vi "mobileye_disp.vi"(11 "x_view":dbl[](array[numeric])=[0.0, 0.5, 1.0, 1.5, 2.0, 2.5, 3.0, 3.5, 4.0, 4.5, 5.0, 5.5, 6.0, 6.5, 7.0, 7.5, 8.0, 8.5, 9.0, 9.5, 10.0, 10.5, 11.0, 11.5, 12.0, 12.5, 13.0, 13.5, 14.0, 14.5, 15.0, 15.5, 16.0, 16.5, 17.0, 17.5, 18.0, 18.5, 19.0, 19.5, 20.0, 20.5, 21.0, 21.5, 22.0, 22.5, 23.0, 23.5, 24.0, 24.5, 25.0, 25.5, 26.0, 26.5, 27.0, 27.5, 28.0, 28.5, 29.0, 29.5, 30.0, 30.5, 31.0, 31.5, 32.0, 32.5, 33.0, 33.5, 34.0, 34.5, 35.0, 35.5, 36.0, 36.5, 37.0, 37.5, 38.0, 38.5, 39.0, 39.5, 40.0, 40.5, 41.0, 41.5, 42.0, 42.5, 43.0, 43.5, 44.0, 44.5, 45.0, 45.5, 46.0, 46.5, 47.0, 47.5, 48.0, 48.5, 49.0, 49.5, 50.0, 50.5, 51.0, 51.5, 52.0, 52.5, 53.0, 53.5, 54.0, 54.5, 55.0, 55.5, 56.0, 56.5, 57.0, 57.5, 58.0, 58.5, 59.0, 59.5, 60.0, 60.5, 61.0, 61.5, 62.0, 62.5, 63.0, 63.5, 64.0, 64.5, 65.0, 65.5, 66.0, 66.5, 67.0, 67.5, 68.0, 68.5, 69.0, 69.5, 70.0, 70.5, 71.0, 71.5, 72.0, 72.5, 73.0, 73.5, 74.0, 74.5, 75.0, 75.5, 76.0, 76.5, 77.0, 77.5, 78.0, 78.5, 79.0, 79.5, 80.0, 80.5, 81.0, 81.5, 82.0, 82.5, 83.0, 83.5, 84.0, 84.5, 85.0, 85.5, 86.0, 86.5, 87.0, 87.5, 88.0, 88.5, 89.0, 89.5, 90.0, 90.5, 91.0, 91.5, 92.0, 92.5, 93.0, 93.5, 94.0, 94.5, 95.0, 95.5, 96.0, 96.5, 97.0, 97.5, 98.0, 98.5, 99.0, 99.5, 100.0, 100.5, 101.0, 101.5, 102.0, 102.5, 103.0, 103.5, 104.0, 104.5, 105.0, 105.5, 106.0, 106.5, 107.0, 107.5, 108.0, 108.5, 109.0, 109.5, 110.0, 110.5, 111.0, 111.5, 112.0, 112.5, 113.0, 113.5, 114.0, 114.5, 115.0, 115.5, 116.0, 116.5, 117.0, 117.5, 118.0, 118.5, 119.0, 119.5, 120.0, 120.5, 121.0, 121.5, 122.0, 122.5, 123.0, 123.5, 124.0, 124.5, 125.0, 125.5, 126.0, 126.5, 127.0, 127.5, 128.0]) -> (3 "XY Graph":cluster{"Y":dbl[], "Y":dbl[]}[](graph)=[{"Y"=[1.82421875, 1.8301353427767753, 1.835194070339203, 1.8394013252854347, 1.8427635002136231, 1.84528698772192, 1.8469781804084777, 1.8478434708714486, 1.8478892517089844, 1.8471219155192375, 1.84554785490036, 1.8431734624505043, 1.8400051307678222, 1.8360492524504661, 1.8313122200965881, 1.8258004263043404, 1.819520263671875, 1.8124781247973443, 1.8046804022789003, 1.796133488714695, 1.7868437767028809, 1.77681765884161, 1.7660615277290344, 1.7545817759633064, 1.742384796142578, 1.7294769808650017, 1.7158647227287291, 1.701554414331913, 1.686552448272705, 1.6708652171492577, 1.654499113559723, 1.637460530102253, 1.619755859375, 1.6013914939761162, 1.5823738265037537, 1.5627092495560646, 1.5424041557312012, 1.5214649376273155, 1.4998979878425598, 1.4777096989750862, 1.4549064636230469, 1.431494674384594, 1.4074807238578795, 1.3828710046410562, 1.3576719093322753, 1.3318898305296898, 1.3055311608314515, 1.2786022928357124, 1.251109619140625, 1.2230595323443412], "Y"=[0.0, 0.5, 1.0, 1.5, 2.0, 2.5, 3.0, 3.5, 4.0, 4.5, 5.0, 5.5, 6.0, 6.5, 7.0, 7.5, 8.0, 8.5, 9.0, 9.5, 10.0, 10.5, 11.0, 11.5, 12.0, 12.5, 13.0, 13.5, 14.0, 14.5, 15.0, 15.5, 16.0, 16.5, 17.0, 17.5, 18.0, 18.5, 19.0, 19.5, 20.0, 20.5, 21.0, 21.5, 22.0, 22.5, 23.0, 23.5, 24.0, 24.5]}, {"Y"=[-1.22265625, -1.2167396572232247, -1.211680929660797, -1.2074736747145653, -1.2041114997863769, -1.20158801227808, -1.1998968195915223, -1.1990315291285514, -1.1989857482910156, -1.1997530844807625, -1.20132714509964, -1.2037015375494957, -1.2068698692321778, -1.2108257475495339, -1.2155627799034119, -1.2210745736956596, -1.227354736328125, -1.2343968752026557, -1.2421945977210997, -1.250741511285305, -1.2600312232971191, -1.27005734115839, -1.2808134722709656, -1.2922932240366936, -1.304490203857422, -1.3173980191349983, -1.3310102772712709, -1.345320585668087, -1.360322551727295, -1.3760097828507423, -1.392375886440277, -1.409414469897747, -1.427119140625, -1.4454835060238838, -1.4645011734962463, -1.4841657504439354, -1.5044708442687988, -1.5254100623726845, -1.5469770121574402, -1.5691653010249138, -1.5919685363769531, -1.615380325615406, -1.6393942761421205, -1.6640039953589438, -1.6892030906677247, -1.7149851694703102, -1.7413438391685485, -1.7682727071642876, -1.795765380859375, -1.8238154676556588, -1.8524165749549866, -1.8815623101592065, -1.911246280670166, -1.9414620938897134, -1.972203357219696, -2.003463678061962, -2.0352366638183597, -2.0675159218907355, -2.1002950596809384, -2.1335676845908162, -2.167327404022217, -2.2015678253769875, -2.2362825560569766, -2.2714652034640315, -2.307109375, -2.3432086780667305, -2.3797567200660703, -2.4167471083998677, -2.4541734504699706, -2.4920293536782263, -2.530308425426483, -2.5690042731165885, -2.6081105041503907, -2.647620725929737, -2.687528545856476, -2.7278275713324547, -2.7685114097595216, -2.809573668539524, -2.8510079550743104, -2.892807876765728, -2.934967041015625, -2.977479055225849, -3.020337526798248, -3.0635360631346704, -3.107068271636963, -3.150927759706974, -3.1951081347465515, -3.2396030041575434, -3.284405975341797, -3.3295106557011604, -3.3749106526374817, -3.4205995735526087, -3.466571025848389, -3.51281861692667, -3.5593359541893004], "Y"=[0.0, 0.5, 1.0, 1.5, 2.0, 2.5, 3.0, 3.5, 4.0, 4.5, 5.0, 5.5, 6.0, 6.5, 7.0, 7.5, 8.0, 8.5, 9.0, 9.5, 10.0, 10.5, 11.0, 11.5, 12.0, 12.5, 13.0, 13.5, 14.0, 14.5, 15.0, 15.5, 16.0, 16.5, 17.0, 17.5, 18.0, 18.5, 19.0, 19.5, 20.0, 20.5, 21.0, 21.5, 22.0, 22.5, 23.0, 23.5, 24.0, 24.5, 25.0, 25.5, 26.0, 26.5, 27.0, 27.5, 28.0, 28.5, 29.0, 29.5, 30.0, 30.5, 31.0, 31.5, 32.0, 32.5, 33.0, 33.5, 34.0, 34.5, 35.0, 35.5, 36.0, 36.5, 37.0, 37.5, 38.0, 38.5, 39.0, 39.5, 40.0, 40.5, 41.0, 41.5, 42.0, 42.5, 43.0, 43.5, 44.0, 44.5, 45.0, 45.5, 46.0, 46.5, 47.0]}, {"Y"=[-0.94, 0.94, 0.94, -0.94, -0.94], "Y"=[-3.2, -3.2, 1.5, 1.5, -3.2]}, {"Y"=[1.984375, 1.978057861328125, 1.9718017578125, 1.965606689453125, 1.95947265625], "Y"=[0.0, 0.5, 1.0, 1.5, 2.0]}, {"Y"=[-5.28125, -5.267578125, -5.25390625, -5.240234375, -5.2265625], "Y"=[0.0, 0.5, 1.0, 1.5, 2.0]}])   [LabVIEW 2015]
uses:
  rio_Global.vi
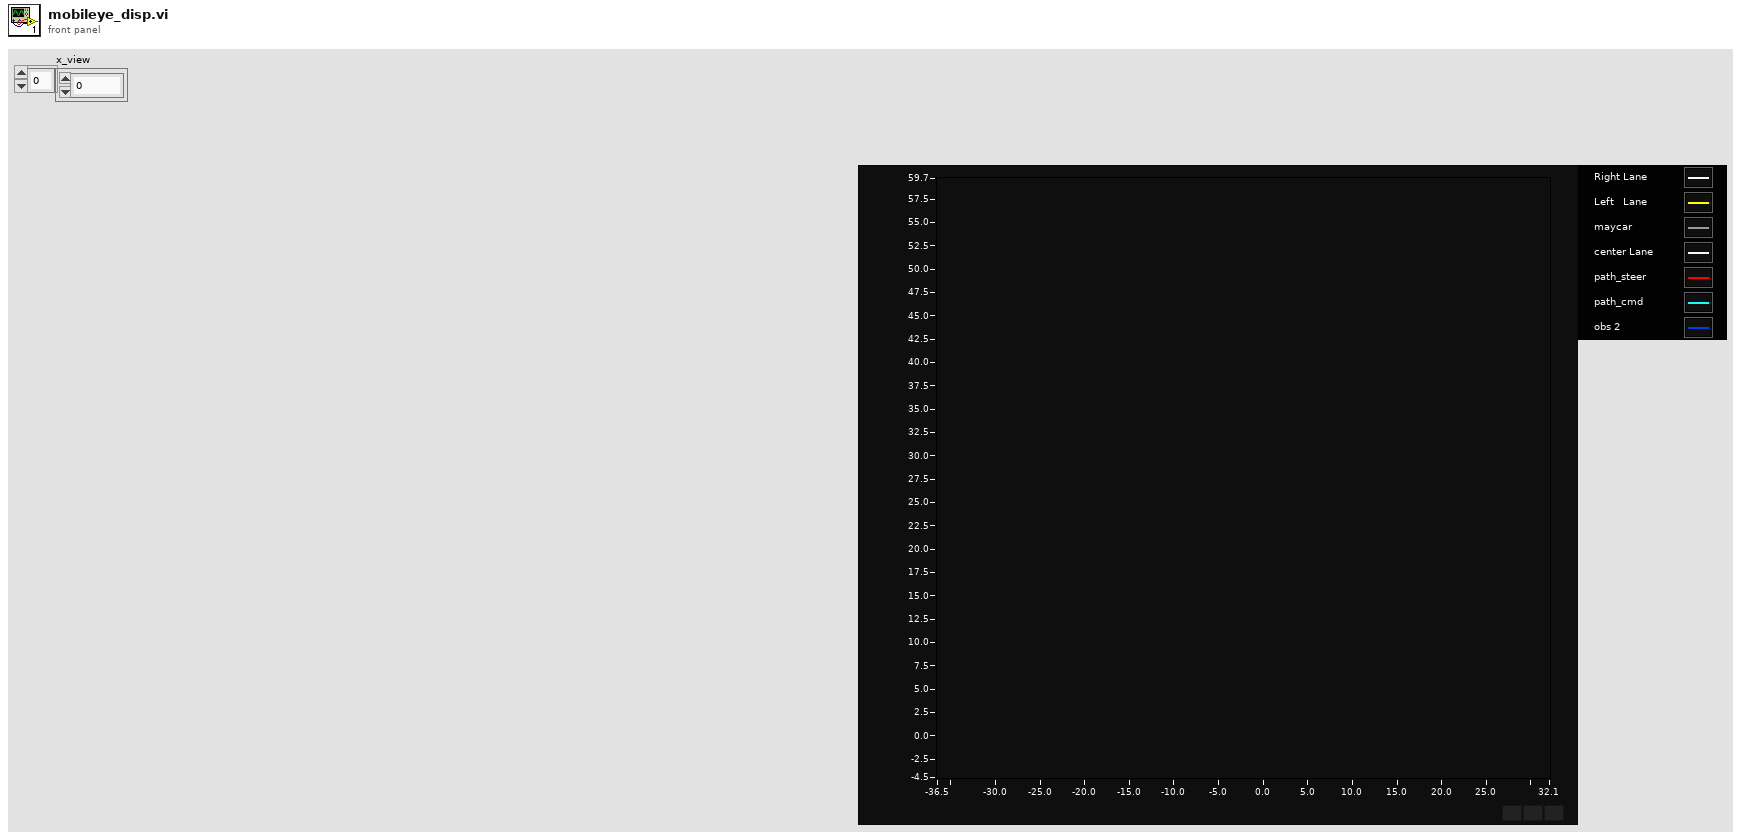
[diagram p1: front panel]
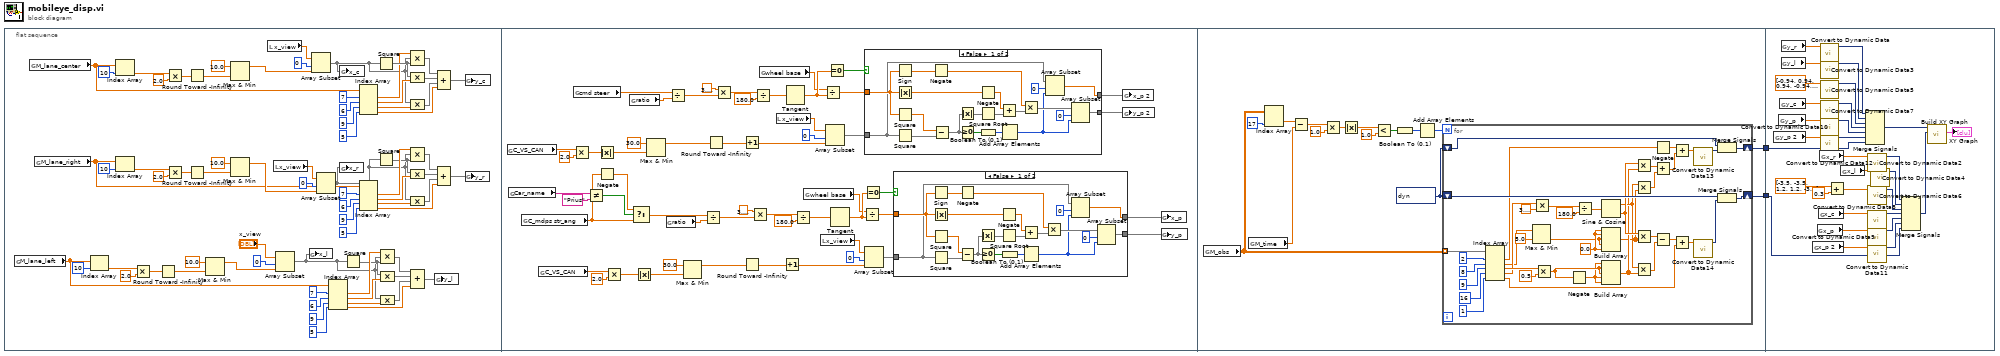
[diagram p0: block diagram]
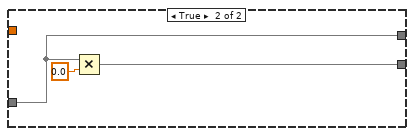
[diagram p2: hidden frame]
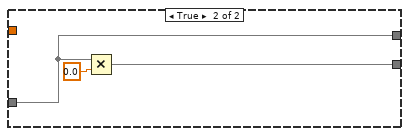
[diagram p3: hidden frame]
diagram:
  n1 = flat-sequence {
    tunnel: [w177] -> w2
    tunnel: [w176] -> w1
    tunnel: w2 -> [w240]
    tunnel: w1 -> [w242]
    frame #0 {
      n2 = global read "rio_Global.vi" "M_lane_left"() -> (w10:dbl[])
      n3 = global read "rio_Global.vi" "M_lane_center"() -> (w12:dbl[])
      n4 = global read "rio_Global.vi" "M_lane_right"() -> (w11:dbl[])
      n5 = Index Array(array=w10, index=10) -> (element=w41:dbl)
      n6 = Index Array(array=w12, index=10) -> (element=w19:dbl)
      n7 = Index Array(array=w11, index=10) -> (element=w49:dbl)
      n8 = Multiply(x=w41, y=2.0) -> (x*y=w42:dbl)
      n9 = Round Toward -Infinity(1:w42) -> (0:w35:dbl)
      n10 = Multiply(x=w19, y=2.0) -> (x*y=w30:dbl)
      n11 = Multiply(x=w49, y=2.0) -> (x*y=w48:dbl)
      n12 = Round Toward -Infinity(1:w30) -> (0:w15:dbl)
      n13 = Round Toward -Infinity(1:w48) -> (0:w39:dbl)
      n14 = Max & Min(x=10.0, y=w35) -> (max(x,y)=w34:dbl)  [unwired: 1 out]
      n15 = Max & Min(x=10.0, y=w15) -> (max(x,y)=w33:dbl)  [unwired: 1 out]
      n16 = Max & Min(x=10.0, y=w39) -> (max(x,y)=w37:dbl)  [unwired: 1 out]
      n17 = local read "x_view"() -> (w18:dbl[])
      n18 = local read "x_view"() -> (w47:dbl[])
      n19 = Array Subset(array="x_view", index=0, length=w34) -> (w4:dbl[])
      n20 = global write "rio_Global.vi" "x_l"(w4) -> ()
      n21 = Array Subset(array=w18, index=0, length=w33) -> (w9:dbl[])
      n22 = Array Subset(array=w47, index=0, length=w37) -> (w6:dbl[])
      n23 = Index Array(array=w10, index #1=7 ("index"), index #2=6 ("index"), index #3=9 ("index"), index #4=5 ("index")) -> (element #1=w54:dbl, element #2=w56:dbl, element #3=w58:dbl, element #4=w62:dbl)
      n24 = global write "rio_Global.vi" "x_c"(w9) -> ()
      n25 = global write "rio_Global.vi" "x_r"(w6) -> ()
      n26 = Square(x=w4) -> (x^2=w52:dbl[])
      n27 = Index Array(array=w12, index #1=7 ("index"), index #2=6 ("index"), index #3=9 ("index"), index #4=5 ("index")) -> (element #1=w13:dbl, element #2=w27:dbl, element #3=w25:dbl, element #4=w32:dbl)
      n28 = Index Array(array=w11, index #1=7 ("index"), index #2=6 ("index"), index #3=9 ("index"), index #4=5 ("index")) -> (element #1=w73:dbl, element #2=w71:dbl, element #3=w69:dbl, element #4=w65:dbl)
      n29 = Square(x=w9) -> (x^2=w21:dbl[])
      n30 = Square(x=w6) -> (x^2=w51:dbl[])
      n31 = Compound Arithmetic op=MULTIPLY(w54, w4, w52) -> (w59:dbl[])
      n32 = Compound Arithmetic op=MULTIPLY(w52, w56) -> (w60:dbl[])
      n33 = Compound Arithmetic op=MULTIPLY(w4, w58) -> (w61:dbl[])
      n34 = Compound Arithmetic op=MULTIPLY(w13, w9, w21) -> (w24:dbl[])
      n35 = Compound Arithmetic op=MULTIPLY(w21, w27) -> (w23:dbl[])
      n36 = Compound Arithmetic op=MULTIPLY(w9, w25) -> (w22:dbl[])
      n37 = Compound Arithmetic op=MULTIPLY(w73, w6, w51) -> (w68:dbl[])
      n38 = Compound Arithmetic op=MULTIPLY(w51, w71) -> (w67:dbl[])
      n39 = Compound Arithmetic op=MULTIPLY(w6, w69) -> (w66:dbl[])
      n40 = Compound Arithmetic op=ADD(w59, w60, w61, w62) -> (w5:dbl[])
      n41 = global write "rio_Global.vi" "y_l"(w5) -> ()
      n42 = Compound Arithmetic op=ADD(w24, w23, w22, w32) -> (w8:dbl[])
      n43 = Compound Arithmetic op=ADD(w68, w67, w66, w65) -> (w7:dbl[])
      n44 = global write "rio_Global.vi" "y_c"(w8) -> ()
      n45 = global write "rio_Global.vi" "y_r"(w7) -> ()
    }
    frame #1 {
      n46 = global read "rio_Global.vi" "C_VS_CAN"() -> (w84:dbl)
      n47 = global read "rio_Global.vi" "Car_name"() -> (w80:string)
      n48 = global read "rio_Global.vi" "C_mdps str_ang"() -> (w76:dbl)
      n49 = global read "rio_Global.vi" "C_VS_CAN"() -> (w83:dbl)
      n50 = Multiply(x=w84, y=2.0) -> (x*y=w103:dbl)
      n51 = global read "rio_Global.vi" "cmd steer"() -> (w93:dbl)
      n52 = Not Equal?(x=w80, y="Prius") -> (x != y?=w78:bool)
      n53 = Absolute Value(x=w103) -> (abs(x)=w104:dbl)
      n54 = Negate(x=w76) -> (-x=w77:dbl)
      n55 = Multiply(x=w83, y=2.0) -> (x*y=w118:dbl)
      n56 = global read "rio_Global.vi" "ratio"() -> (w92:dbl)
      n57 = Select(t=w77, s=w78, f=w76) -> (s? t:f=w75:dbl)
      n58 = Absolute Value(x=w118) -> (abs(x)=w117:dbl)
      n59 = Max & Min(x=30.0, y=w104) -> (max(x,y)=w105:dbl)  [unwired: 1 out]
      n60 = global read "rio_Global.vi" "ratio"() -> (w91:dbl)
      n61 = Divide(x=w93, y=w92) -> (x/y=w109:dbl)
      n62 = Max & Min(x=30.0, y=w117) -> (max(x,y)=w116:dbl)  [unwired: 1 out]
      n63 = Divide(x=w75, y=w91) -> (x/y=w112:dbl)
      n64 = Round Toward -Infinity(1:w105) -> (0:w100:dbl)
      n65 = Multiply(x=3.141592653589793, y=w109) -> (x*y=w95:dbl)
      n66 = Increment(x=w100) -> (x+1=w102:dbl)
      n67 = Round Toward -Infinity(1:w116) -> (0:w121:dbl)
      n68 = Multiply(x=3.141592653589793, y=w112) -> (x*y=w126:dbl)
      n69 = Divide(x=w95, y=180.0) -> (x/y=w97:dbl)
      n70 = global read "rio_Global.vi" "wheel base"() -> (w90:dbl)
      n71 = local read "x_view"() -> (w98:dbl[])
      n72 = Increment(x=w121) -> (x+1=w119:dbl)
      n73 = Tangent(1:w97) -> (0:w107:dbl)
      n74 = Divide(x=w126, y=180.0) -> (x/y=w124:dbl)
      n75 = global read "rio_Global.vi" "wheel base"() -> (w89:dbl)
      n76 = local read "x_view"() -> (w123:dbl[])
      n77 = Divide(x=w90, y=w107) -> (x/y=w81:dbl)
      n78 = Array Subset(array=w98, index=0, length=w102) -> (w108:dbl[])
      n79 = Equal To 0?(x=w107) -> (x = 0?=w110:bool)
      n80 = Tangent(1:w124) -> (0:w114:dbl)
      n81 = Divide(x=w89, y=w114) -> (x/y=w82:dbl)
      n82 = Equal To 0?(x=w114) -> (x = 0?=w111:bool)
      n83 = case shown="False" w110 {
        tunnel: w81 -> [w143 _]
        tunnel: [w133 w148] -> w86
        tunnel: w108 -> [w131 w150]
        tunnel: [w129 w150] -> w85
        frame False {
          n84 = Square(x=w143) -> (x^2=w147:dbl)
          n85 = Square(x=w131) -> (x^2=w139:dbl[])
          n86 = Sign(1:w143) -> (0:w142:dbl)
          n87 = Absolute Value(x=w143) -> (abs(x)=w145:dbl)
          n88 = Negate(x=w142) -> (-x=w141:dbl)
          n89 = Subtract(x=w147, y=w139) -> (x-y=w137:dbl[])
          n90 = Absolute Value(x=w137) -> (abs(x)=w146:dbl[])
          n91 = Greater Or Equal To 0?(x=w137) -> (x >= 0?=w136:bool[])
          n92 = Negate(x=w145) -> (-x=w144:dbl)
          n93 = Square Root(x=w146) -> (sqrt(x)=w138:dbl[])
          n94 = Boolean To (0,1)(Boolean=w136) -> (0, 1=w135:i16[])
          n95 = Add(x=w144, y=w138) -> (x+y=w140:dbl[])
          n96 = Add Array Elements(numeric array=w135) -> (sum=w130:i16)
          n97 = Multiply(x=w141, y=w140) -> (x*y=w134:dbl[])
          n98 = Array Subset(array=w131, index=0, length=w130) -> (w129:dbl[])
          n99 = Array Subset(array=w134, index=0, length=w130) -> (w133:dbl[])
        }
        frame True {
          n100 = Multiply(x=w150, y=0.0) -> (x*y=w148:dbl[])
        }
      }
      n101 = Array Subset(array=w123, index=0, length=w119) -> (w113:dbl[])
      n102 = case shown="False" w111 {
        tunnel: w82 -> [w166 _]
        tunnel: [w156 w171] -> w87
        tunnel: w113 -> [w154 w173]
        tunnel: [w152 w173] -> w88
        frame False {
          n103 = Square(x=w166) -> (x^2=w170:dbl)
          n104 = Square(x=w154) -> (x^2=w162:dbl[])
          n105 = Sign(1:w166) -> (0:w165:dbl)
          n106 = Absolute Value(x=w166) -> (abs(x)=w168:dbl)
          n107 = Negate(x=w165) -> (-x=w164:dbl)
          n108 = Subtract(x=w170, y=w162) -> (x-y=w160:dbl[])
          n109 = Absolute Value(x=w160) -> (abs(x)=w169:dbl[])
          n110 = Greater Or Equal To 0?(x=w160) -> (x >= 0?=w159:bool[])
          n111 = Negate(x=w168) -> (-x=w167:dbl)
          n112 = Square Root(x=w169) -> (sqrt(x)=w161:dbl[])
          n113 = Boolean To (0,1)(Boolean=w159) -> (0, 1=w158:i16[])
          n114 = Add(x=w167, y=w161) -> (x+y=w163:dbl[])
          n115 = Add Array Elements(numeric array=w158) -> (sum=w153:i16)
          n116 = Multiply(x=w164, y=w163) -> (x*y=w157:dbl[])
          n117 = Array Subset(array=w154, index=0, length=w153) -> (w152:dbl[])
          n118 = Array Subset(array=w157, index=0, length=w153) -> (w156:dbl[])
        }
        frame True {
          n119 = Multiply(x=w173, y=0.0) -> (x*y=w171:dbl[])
        }
      }
      n120 = global write "rio_Global.vi" "x_p 2"(w85) -> ()
      n121 = global write "rio_Global.vi" "y_p 2"(w86) -> ()
      n122 = global write "rio_Global.vi" "x_p"(w88) -> ()
      n123 = global write "rio_Global.vi" "y_p"(w87) -> ()
    }
    frame #2 {
      w179 = dynamicdata [] ("Dynamic Data Type")
      n124 = global read "rio_Global.vi" "M_obs"() -> (w175:dbl[][])
      n125 = global read "rio_Global.vi" "M_time"() -> (w174:dbl)
      n126 = Index Array(array=w175, index (col)=17 ("disabled index (col)")) -> (element=w187:dbl[])  [unwired: 1 in]
      n127 = Subtract(x=w187, y=w174) -> (x-y=w186:dbl[])
      n128 = Multiply(x=w186, y=1.0) -> (x*y=w184:dbl[])
      n129 = Absolute Value(x=w184) -> (abs(x)=w183:dbl[])
      n130 = Less?(x=w183, y=1.0) -> (x < y?=w181:bool[])
      n131 = Boolean To (0,1)(Boolean=w181) -> (0, 1=w180:i16[])
      n132 = Add Array Elements(numeric array=w180) -> (sum=w178:i16)
      n133 = for {
        N: w178 -> [_]
        tunnel: w175 -> [w228] mode=indexing
        shift-right: [w214] -> w177
        shift-left: w179 -> [w216]
        shift-right: [w212] -> w176
        shift-left: w179 -> [w211]
        w204 = 0.0 ("element")
        n134 = Index Array(array=w228, index #1=2 ("index"), index #2=8 ("index"), index #3=9 ("index"), index #4=16 ("index"), index #5=1 ("index")) -> (element #1=w207:dbl, element #2=w203:dbl, element #3=w225:dbl, element #4=w220:dbl, element #5=w208:dbl)
        n135 = Max & Min(x=w203, y=5.0) -> (min(x,y)=w201:dbl)  [unwired: 1 out]
        n136 = Multiply(x=w220, y=3.141592653589793) -> (x*y=w218:dbl)
        n137 = Multiply(x=w225, y=0.5) -> (x*y=w223:dbl)
        n138 = Negate(x=w223) -> (-x=w222:dbl)
        n139 = Divide(x=w218, y=180.0) -> (x/y=w192:dbl)
        n140 = Sine & Cosine(0:w192) -> (1:w196:dbl, 2:w197:dbl)
        n141 = Build Array(w204, w204, w201, w201, w204) -> (w191:dbl[])
        n142 = Build Array(w222, w223, w223, w222, w222) -> (w193:dbl[])
        n143 = Multiply(x=w197, y=w193) -> (x*y=w194:dbl[])
        n144 = Multiply(x=w196, y=w191) -> (x*y=w195:dbl[])
        n145 = Multiply(x=w197, y=w191) -> (x*y=w198:dbl[])
        n146 = Multiply(x=w196, y=w193) -> (x*y=w199:dbl[])
        n147 = Negate(x=w207) -> (-x=w206:dbl)
        n148 = Add(x=w194, y=w195) -> (x+y=w190:dbl[])
        n149 = Subtract(x=w198, y=w199) -> (x-y=w189:dbl[])
        n150 = Add(x=w206, y=w190) -> (x+y=w205:dbl[])
        n151 = Add(x=w189, y=w208) -> (x+y=w210:dbl[])
        n152 = call "Convert to Dynamic Data13"("Array"=w205) -> ("Dynamic Data Type"=w215:dynamicdata)  [unwired: 3 in]
        n153 = call "Convert to Dynamic Data14"("Array"=w210) -> ("Dynamic Data Type"=w213:dynamicdata)  [unwired: 3 in]
        n154 = Merge Signals(w216, w215) -> (w214:dynamicdata)
        n155 = Merge Signals(w211, w213) -> (w212:dynamicdata)
      }
    }
    frame #3 {
      n156 = global read "rio_Global.vi" "y_p 2"() -> (w234:dbl[])
      n157 = global read "rio_Global.vi" "y_p"() -> (w235:dbl[])
      n158 = global read "rio_Global.vi" "y_c"() -> (w236:dbl[])
      n159 = global read "rio_Global.vi" "y_r"() -> (w238:dbl[])
      n160 = global read "rio_Global.vi" "y_l"() -> (w237:dbl[])
      n161 = global read "rio_Global.vi" "x_p 2"() -> (w229:dbl[])
      n162 = global read "rio_Global.vi" "x_p"() -> (w230:dbl[])
      n163 = global read "rio_Global.vi" "x_c"() -> (w231:dbl[])
      n164 = global read "rio_Global.vi" "x_r"() -> (w233:dbl[])
      n165 = call "Convert to Dynamic Data"("Array"=w238) -> ("Dynamic Data Type"=w259:dynamicdata)  [unwired: 3 in]
      n166 = call "Convert to Dynamic Data3"("Array"=w237) -> ("Dynamic Data Type"=w256:dynamicdata)  [unwired: 3 in]
      n167 = call "Convert to Dynamic Data5"("Array"=dbl[] [-0.94, 0.94, 0.94, -0.94, -0.94] ("appended array 2")) -> ("Dynamic Data Type"=w251:dynamicdata)  [unwired: 3 in]
      n168 = call "Convert to Dynamic Data7"("Array"=w236) -> ("Dynamic Data Type"=w246:dynamicdata)  [unwired: 3 in]
      n169 = call "Convert to Dynamic Data10"("Array"=w235) -> ("Dynamic Data Type"=w243:dynamicdata)  [unwired: 3 in]
      n170 = call "Convert to Dynamic Data12"("Array"=w234) -> ("Dynamic Data Type"=w239:dynamicdata)  [unwired: 3 in]
      n171 = Add(x=dbl[] [-3.5, -3.5, 1.2, 1.2, -3.5] ("appended array"), y=0.3) -> (x+y=w248:dbl[])
      n172 = global read "rio_Global.vi" "x_l"() -> (w232:dbl[])
      n173 = Merge Signals(w259, w256, w251, w246, w243, w239, w240) -> (w253:dynamicdata)
      n174 = call "Convert to Dynamic Data2"("Array"=w233) -> ("Dynamic Data Type"=w258:dynamicdata)  [unwired: 3 in]
      n175 = call "Convert to Dynamic Data6"("Array"=w248) -> ("Dynamic Data Type"=w250:dynamicdata)  [unwired: 3 in]
      n176 = call "Convert to Dynamic Data8"("Array"=w231) -> ("Dynamic Data Type"=w245:dynamicdata)  [unwired: 3 in]
      n177 = call "Convert to Dynamic Data9"("Array"=w230) -> ("Dynamic Data Type"=w244:dynamicdata)  [unwired: 3 in]
      n178 = call "Convert to Dynamic Data11"("Array"=w229) -> ("Dynamic Data Type"=w241:dynamicdata)  [unwired: 3 in]
      n179 = call "Convert to Dynamic Data4"("Array"=w232) -> ("Dynamic Data Type"=w254:dynamicdata)  [unwired: 3 in]
      n180 = Merge Signals(w258, w254, w250, w245, w244, w241, w242) -> (w255:dynamicdata)
      n181 = call "Build XY Graph"("Y Input"=w255, "X Input"=w253) -> ("XY Graph"=→"XY Graph":cluster{"X":dbl[], "Y":dbl[]}[])  [unwired: 8 in, 1 out]
    }
  }
